vi "LoadCounterCfg.vi"() -> (3 "Variant":variant)   [LabVIEW 2017, in "NEVSTOP QD Shortcuts.lvlib"]
uses:
  NEVSTOP QD Shortcuts.lvlib
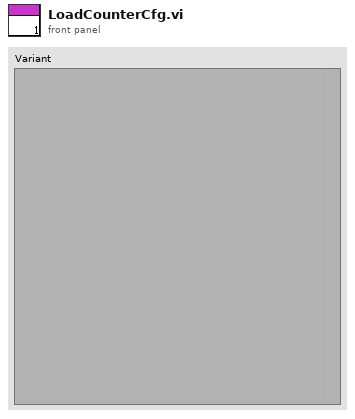
[diagram p1: front panel]
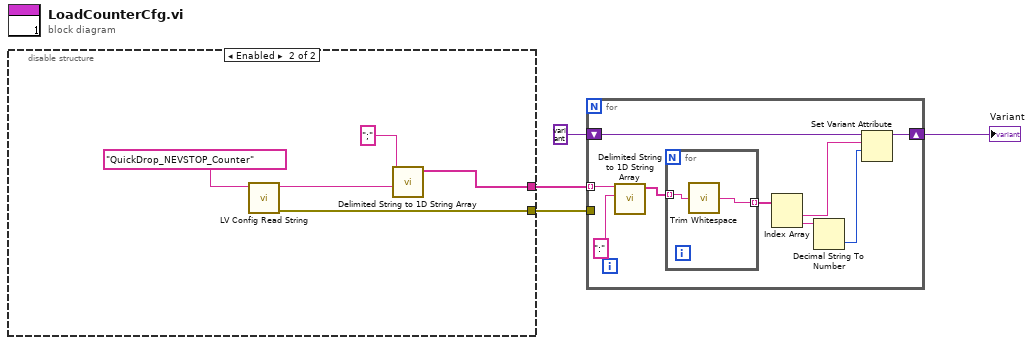
[diagram p0: block diagram]
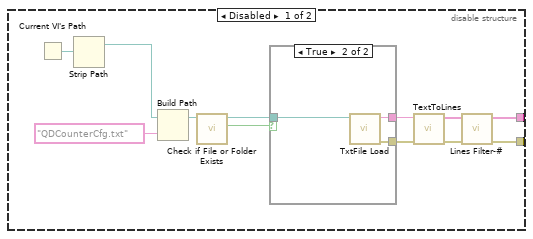
[diagram p2: hidden frame]
diagram:
  n1 = disable-structure shown="Enabled" {
    disable-tunnel: [w9 w20] -> w3
    disable-tunnel: [w8 w23] -> w2
    frame Disabled {
      n2 = Current VI's Path() -> (path=w6:path)
      n3 = Strip Path(path=w6) -> (stripped path=w5:path)  [unwired: 1 out]
      n4 = Build Path(base path=w5, name or relative path="QDCounterCfg.txt") -> (appended path=w14:path)
      n5 = call <vilib>:"Check if File or Folder Exists.vi"("path"=w14) -> ("file or folder exists?"=w7:bool, "dup path"=w16:path)  [unwired: 8 in, 1 out]
      n6 = case shown="True" w7 {
        tunnel: w16 -> [_ w19]
        tunnel: [_ w18] -> w13
        tunnel: [_ w17] -> w12
        frame False {
        }
        frame True {
          n7 = call "TxtFile Load.vi"("Path"=w19) -> ("error out"=w18:errorcluster, "text"=w17:string)  [unwired: 9 in]
        }
      }
      n8 = call "TextToLines.vi"("error in (no error)"=w13, "string"=w12) -> ("error out"=w11:errorcluster, "Lines"=w10:string[])  [unwired: 8 in]
      n9 = call "Lines Filter-#.vi"("error in (no error)"=w11, "Lines"=w10) -> ("error out"=w8:errorcluster, "Config Text List"=w9:string[])  [unwired: 8 in]
    }
    frame Enabled {
      n10 = call <resource>:"LV Config Read String.vi"("key"="QuickDrop_NEVSTOP_Counter") -> ("error out"=w23:errorcluster, "value"=w22:string)  [unwired: 4 in, 1 out]
      n11 = call "Delimited String to 1D String Array.vi"("delimiter"=w22, "delimited string"=";" ("delimiter (Tab)")) -> ("string array"=w20:string[])  [unwired: 9 in]
    }
  }
  n12 = for {
    tunnel: w3 -> [w25] mode=indexing
    tunnel: w2 -> [_]
    shift-right: [w32] -> w4
    shift-left: variant ("Variant") -> [w31]
    n13 = call "Delimited String to 1D String Array.vi"("delimiter"=":" ("delimiter (Tab)"), "delimited string"=w25) -> ("string array"=w33:string[])  [unwired: 9 in]
    n14 = for {
      tunnel: w33 -> [w35] mode=indexing
      tunnel: [w34] -> w30 mode=indexing
      n15 = call-poly <vilib>:"Trim Whitespace.vi"("string"=w35) -> ("trimmed string"=w34:string)  [unwired: 1 in]
    }
    n16 = Index Array(array=w30) -> (element #1=w29:string, element #2=w28:string)  [unwired: 2 in]
    n17 = Decimal String To Number(string=w28) -> (number=w27:i32)  [unwired: 2 in, 1 out]
    n18 = Set Variant Attribute(Variant=w31, name=w29, value=w27) -> (Variant out=w32:variant)  [unwired: 1 in, 2 out]
  }
  "Variant" <- w4
